vi "test Loopback Timestamp with Start and Stop.vi"(8 "error in":errorcluster, 11 "TestCase in":refnum<class "Loopback.lvclass">) -> (0 "error out":errorcluster, 3 "TestCase out":refnum<class "Loopback.lvclass">)   [LabVIEW 2020, in "Loopback.lvclass"]
uses:
  Loopback.lvclass
  C:/dev/niveristand-custom-device-testing-tools/VeriStandTestCase/VeriStandTestCase.lvclass
  485b7c2b-8320-4722-9ec7-d01f27c65546.vi
  94b1695b-f377-4b7f-b0ef-3ed20e67d1fe.vi
  <vilib>/NI VeriStand/Execution/Workspace/NI VeriStand - Get Single Channel Value.vi
  <vilib>/NI VeriStand/Execution/Workspace/NI VeriStand - Get Multiple Channel Values.vi
  <vilib>/addons/_JKI Toolkits/VI Tester/TestCase.llb/TestCase.lvclass
  <vilib>/NI VeriStand/Execution/Workspace/NI_VS Workspace ExecutionAPI.lvlib
  0501850f-2cfc-4d6c-aa4b-93a987d0c38c.vi
  6667ace5-0e9a-4c06-9531-f483ffd5813a.vi
  <vilib>/NI VeriStand/Execution/Workspace/NI VeriStand - Set Single Channel Value.vi
  4e80fba6-9357-4824-b8af-6da14ea03a7c.vi
  C:/Program Files (x86)/National Instruments/LabVIEW 2020/vi.lib/addons/_JKI Toolkits/VI Tester/TestCase.llb/TestCase.lvclass
  C:/dev/niveristand-ballard-milStd1553-custom-device/Source/Custom Device Support/Tests/System/Loopback/Loopback.lvclass
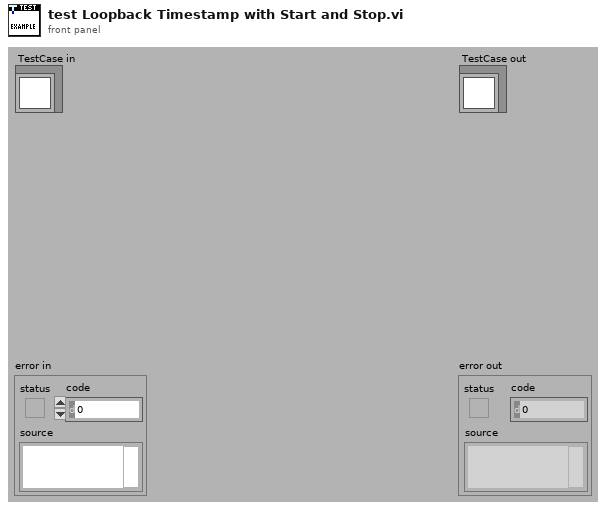
[diagram p1: front panel]
types:
  T1 = typedef "NI_VS Workspace ExecutionAPI.lvlib/WorkspaceAPI.ctl" = refnum<k24>
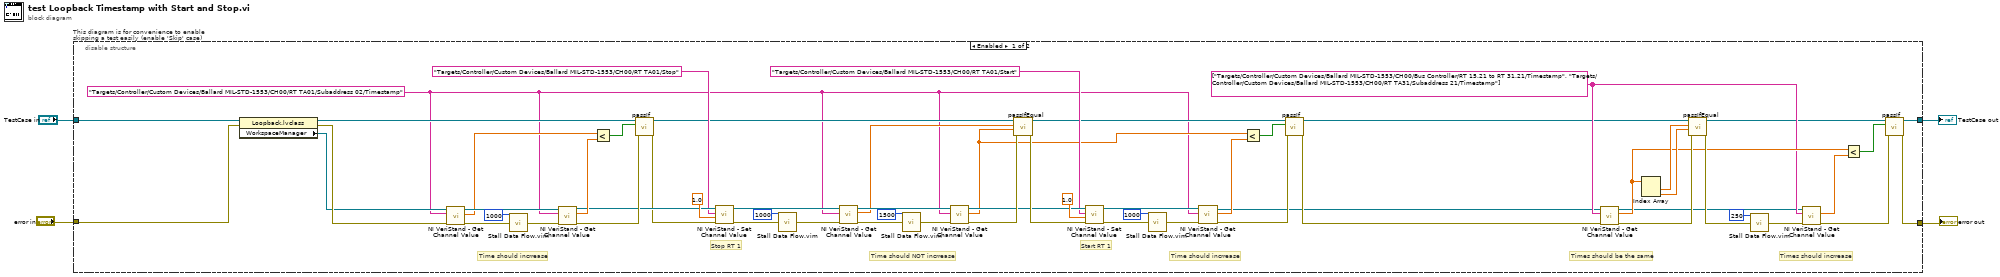
[diagram p0: block diagram]
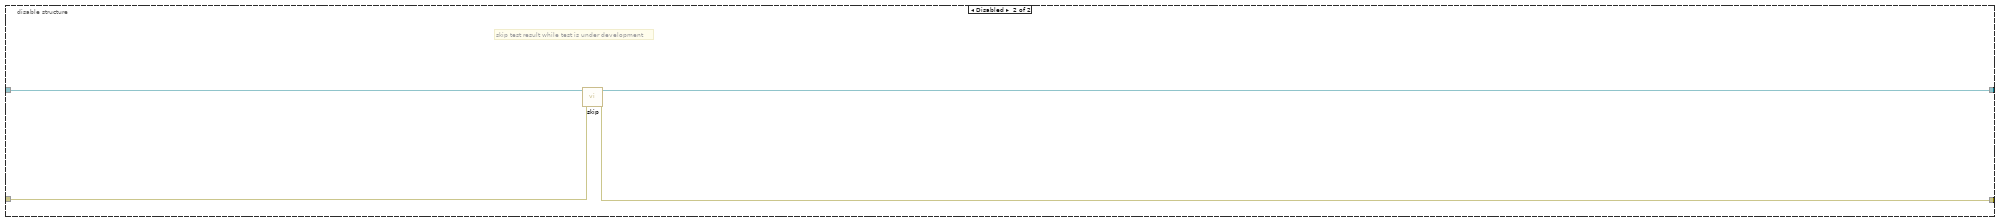
[diagram p2: hidden frame]
diagram:
  n1 = disable-structure "This diagram is for convenience to enable skipping a test easily (enable 'Skip' case)" shown="Enabled" {
    disable-tunnel: "TestCase in" -> [w56 w68]
    disable-tunnel: [w37 w67] -> w1
    disable-tunnel: [w43 w66] -> w3
    disable-tunnel: "error in" -> [w55 w65]
    frame Enabled {
      w40 = string[] ["Targets/Controller/Custom Devices/Ballard MIL-STD-1553/CH00/Bus Controller/RT 15.21 to RT 31.21/Timestamp", "Targets/Controller/Custom Devices/Ballard MIL-STD-1553/CH00/RT TA31/Subaddress 21/Timestamp"] ("Channels")
      w5 = "Targets/Controller/Custom Devices/Ballard MIL-STD-1553/CH00/RT TA01/Subaddress 02/Timestamp"
      # "Time should incrrease"
      # "Start RT 1"
      # "Time should NOT incrrease"
      # "Stop RT 1"
      # "Times should incrrease"
      # "Times should be the same"
      # "Time should incrrease"
      n2 = property class="Loopback.lvclass"(reference=w56, error in=w55) -> (reference out=w64:refnum<class "Loopback.lvclass">, error out=w59:errorcluster, "WorkspaceManager"=w57:T1)
      n3 = call-poly <vilib>:"NI VeriStand - Get Channel Value.vi"("error in (no error)"=w59, "Channel"=w5, "WorkspaceManager in"=w57) -> ("error out"=w61:errorcluster, "Value"=w53:dbl, "WorkspaceManager out"=w63:T1)  [unwired: 6 in]
      n4 = call "Stall Data Flow.vim"("value in"=w61, "milliseconds to wait"=u32 1000) -> ("value out"=w62:errorcluster)  [unwired: 1 out]
      n5 = call-poly <vilib>:"NI VeriStand - Get Channel Value.vi"("error in (no error)"=w62, "Channel"=w5, "WorkspaceManager in"=w63) -> ("error out"=w58:errorcluster, "Value"=w52:dbl, "WorkspaceManager out"=w33:T1)  [unwired: 6 in]
      n6 = Less?(x=w53, y=w52) -> (x < y?=w51:bool)
      n7 = call-dynamic "passIf.vi"("error in (no error)"=w58, "pass"=w51, "TestCase in"=w64) -> ("error out"=w31:errorcluster, "TestCase out"=w24:refnum<class "Loopback.lvclass">)  [unwired: 7 in]
      n8 = call-poly <vilib>:"NI VeriStand - Set Channel Value.vi"("error in (no error)"=w31, "Value"=1.0, "Channel"="Targets/Controller/Custom Devices/Ballard MIL-STD-1553/CH00/RT TA01/Stop", "WorkspaceManager in"=w33) -> ("error out"=w35:errorcluster, "WorkspaceManager out"=w28:T1)  [unwired: 6 in]
      n9 = call "Stall Data Flow.vim"("value in"=w35, "milliseconds to wait"=u32 1000) -> ("value out"=w27:errorcluster)  [unwired: 1 out]
      n10 = call-poly <vilib>:"NI VeriStand - Get Channel Value.vi"("error in (no error)"=w27, "Channel"=w5, "WorkspaceManager in"=w28) -> ("error out"=w29:errorcluster, "Value"=w23:dbl, "WorkspaceManager out"=w26:T1)  [unwired: 6 in]
      n11 = call "Stall Data Flow.vim"("value in"=w29, "milliseconds to wait"=u32 1500) -> ("value out"=w25:errorcluster)  [unwired: 1 out]
      n12 = call-poly <vilib>:"NI VeriStand - Get Channel Value.vi"("error in (no error)"=w25, "Channel"=w5, "WorkspaceManager in"=w26) -> ("error out"=w22:errorcluster, "Value"=w11:dbl, "WorkspaceManager out"=w16:T1)  [unwired: 6 in]
      n13 = call-dynamic "passIfEqual.vi"("error in (no error)"=w22, "y"=w11, "x"=w23, "TestCase in"=w24) -> ("error out"=w17:errorcluster, "TestCase out"=w10:refnum<class "Loopback.lvclass">)  [unwired: 6 in]
      n14 = call-poly <vilib>:"NI VeriStand - Set Channel Value.vi"("error in (no error)"=w17, "Value"=1.0, "Channel"="Targets/Controller/Custom Devices/Ballard MIL-STD-1553/CH00/RT TA01/Start", "WorkspaceManager in"=w16) -> ("error out"=w19:errorcluster, "WorkspaceManager out"=w21:T1)  [unwired: 6 in]
      n15 = call "Stall Data Flow.vim"("value in"=w19, "milliseconds to wait"=u32 1000) -> ("value out"=w14:errorcluster)  [unwired: 1 out]
      n16 = call-poly <vilib>:"NI VeriStand - Get Channel Value.vi"("error in (no error)"=w14, "Channel"=w5, "WorkspaceManager in"=w21) -> ("error out"=w9:errorcluster, "Value"=w12:dbl, "WorkspaceManager out"=w7:T1)  [unwired: 6 in]
      n17 = Less?(x=w11, y=w12) -> (x < y?=w13:bool)
      n18 = call-dynamic "passIf.vi"("error in (no error)"=w9, "pass"=w13, "TestCase in"=w10) -> ("error out"=w8:errorcluster, "TestCase out"=w6:refnum<class "Loopback.lvclass">)  [unwired: 7 in]
      n19 = call-poly <vilib>:"NI VeriStand - Get Channel Value.vi"("error in (no error)"=w8, "Channels"=w40, "WorkspaceManager in"=w7) -> ("error out"=w54:errorcluster, "Values"=w42:dbl[], "WorkspaceManager out"=w39:T1)  [unwired: 6 in]
      n20 = Index Array(array=w42) -> (element #1=w50:dbl, element #2=w49:dbl)  [unwired: 2 in]
      n21 = call-dynamic "passIfEqual.vi"("error in (no error)"=w54, "y"=w49, "x"=w50, "TestCase in"=w6) -> ("error out"=w48:errorcluster, "TestCase out"=w38:refnum<class "Loopback.lvclass">)  [unwired: 6 in]
      n22 = call "Stall Data Flow.vim"("value in"=w48, "milliseconds to wait"=u32 250) -> ("value out"=w46:errorcluster)  [unwired: 1 out]
      n23 = call-poly <vilib>:"NI VeriStand - Get Channel Value.vi"("error in (no error)"=w46, "Channels"=w40, "WorkspaceManager in"=w39) -> ("error out"=w44:errorcluster, "Values"=w41:dbl[])  [unwired: 6 in, 1 out]
      n24 = Less?(x=w42, y=w41) -> (x < y?=w45:bool)
      n25 = call-dynamic "passIf.vi"("error in (no error)"=w44, "pass"=w45, "TestCase in"=w38) -> ("error out"=w43:errorcluster, "TestCase out"=w37:refnum<class "Loopback.lvclass">)  [unwired: 7 in]
    }
    frame Disabled {
      # "skip test result while test is under development"
      n26 = call <vilib>:"skip.vi"("error in (no error)"=w65, "TestCase in"=w68) -> ("error out"=w66:errorcluster, "TestCase out"=w67:refnum<class "Loopback.lvclass">)  [unwired: 8 in]
    }
  }
  "error out" <- w3
  "TestCase out" <- w1
